vi "Stop.vi"(8 "error in":errorcluster, 11 "WaveformTask in":refnum<class "WaveformTask.lvclass">) -> (0 "error out":errorcluster, 3 "Task out":refnum<class "WaveformTask.lvclass">)   [LabVIEW 2015, in "WaveformTask.lvclass"]
uses:
  WaveformTask.lvclass
  WaveformTask.lvclass/WaveformTask.ctl
  <vilib>/NI/cRIO Wfm/ErrorSelector.ctl
  <vilib>/Utility/error.llb/Error Cluster From Error Code.vi
  <vilib>/rvi/errors/niLvFpgaAdjustHostInterfaceError.vi
  <vilib>/rvi/interface/nirviMethod/nirviMethod.xnode
  DataFIFOs.ctl
  <vilib>/NI/cRIO Wfm/cRIO Wfm.lvlib
  <vilib>/FPGAPlugInAG/Dynamic/niLvFpga_ReadFifo_Dynamic.vi
  <vilib>/rvi/errors/niLvFpgaMergeErrorWithErrorCode.vi
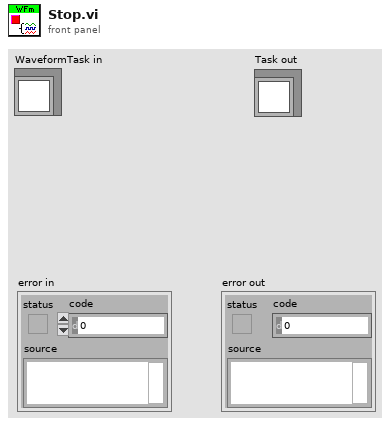
[diagram p1: front panel]
types:
  T1 = typedef "WaveformTask.lvclass/DataFIFOs.ctl" = refnum<k20>
  T2 = typedef "cRIO Wfm.lvlib/ErrorSelector.ctl" = enum16{"Read Timeout", "Module Underflow", "DMA Overflow", "Chan Count", "Run Timeout", "Start Timeout", "Stop Timeout"}
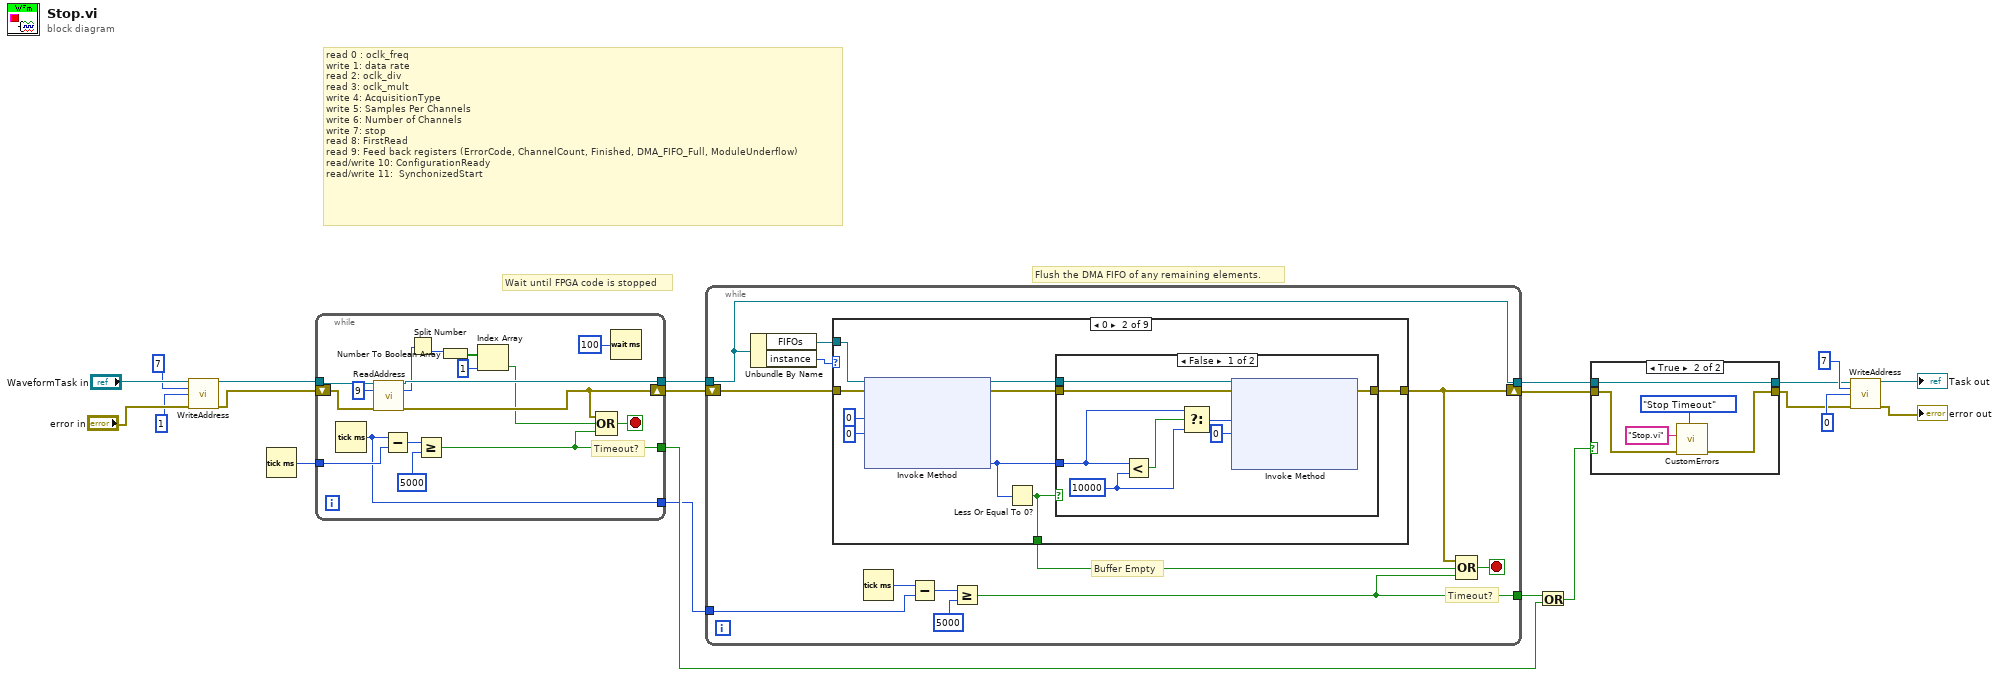
[diagram p0: block diagram]
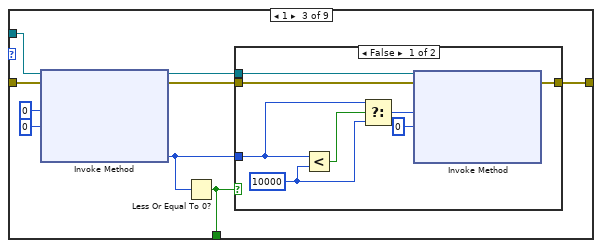
[diagram p4: hidden frame]
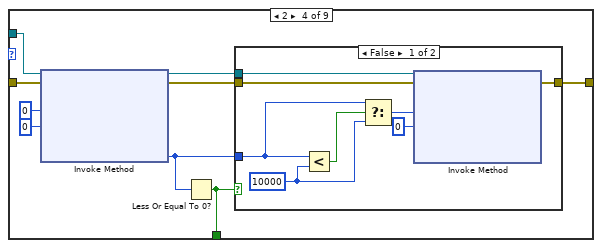
[diagram p6: hidden frame]
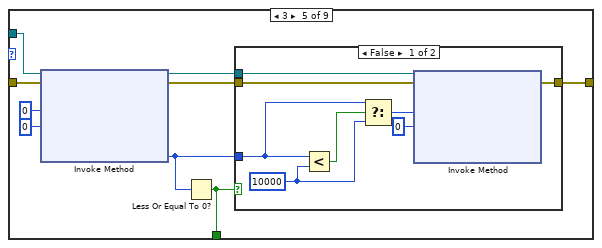
[diagram p8: hidden frame]
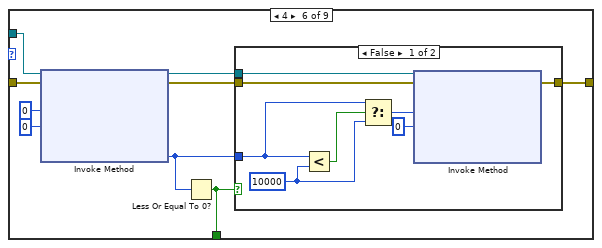
[diagram p10: hidden frame]
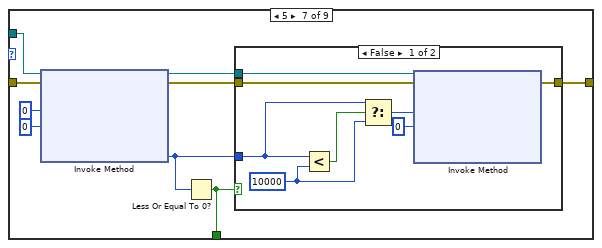
[diagram p12: hidden frame]
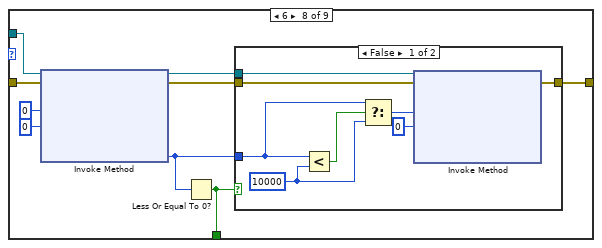
[diagram p14: hidden frame]
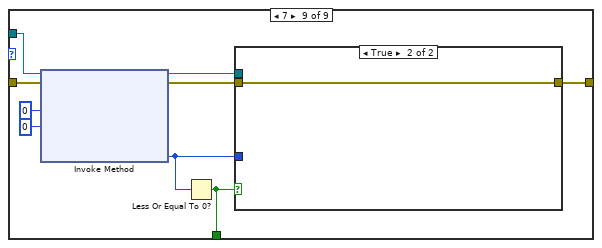
[diagram p16: hidden frame]
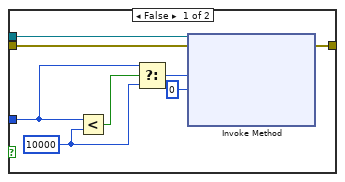
[diagram p17: hidden frame]
diagram:
  # "read 0 : oclk_freq\nwrite 1: data rate\nread 2: oclk_div\nread 3: oclk_mult\nwrite 4: AcquisitionType\nwrite 5: Samples Per Channels\nwrite 6: Number of Channels\nwrite 7: stop\nread 8: FirstRead\nread 9: Feed back registers (ErrorCode, ChannelCount, Finished, DMA_FIFO_Full, ModuleUnderflow)\nread/write 10: ConfigurationReady\nread/write 11:  SynchonizedStart"
  # "Wait until FPGA code is stopped"
  # "Flush the DMA FIFO of any remaining elements."
  n1 = call "WriteAddress.vi"("Task in"="WaveformTask in", "address"=u64 7, "data"=u64 1, "error in (no error)"="error in") -> ("Task out"=w7:refnum<class "WaveformTask.lvclass">, "error out"=w8:errorcluster)  [unwired: 10 in]
  n2 = Tick Count (ms)() -> (millisecond timer value=w17:u32)
  n3 = while {
    tunnel: w7 -> [w31]
    tunnel: [w29] -> w21
    tunnel: w17 -> [w37]
    tunnel: [w33] -> w15
    tunnel: [w32] -> w13
    shift-right: [w27] -> w20
    shift-left: w8 -> [w30]
    stop <- w34 stop-if-true
    # "Timeout?"
    n4 = Tick Count (ms)() -> (millisecond timer value=w32:u32)
    n5 = call "ReadAddress.vi"("Task in"=w31, "address"=u64 9, "error in (no error)"=w30) -> ("Task out"=w29:refnum<class "WaveformTask.lvclass">, "data"=w26:u64, "error out"=w27:errorcluster)  [unwired: 10 in]
    n6 = Subtract(x=w32, y=w37) -> (x-y=w36:u32)
    n7 = Split Number(x=w26) -> (lo(x)=w25:u32)  [unwired: 1 out]
    n8 = Greater Or Equal?(x=w36, y=u32 5000) -> (x >= y?=w33:bool)
    n9 = Number To Boolean Array(number=w25) -> (Boolean array=w24:bool[])
    n10 = Index Array(array=w24, index=1) -> (element=w22:bool)
    n11 = Compound Arithmetic op=OR(w27, w22, w33) -> (w34:bool)
    n12 = Wait (ms)(milliseconds to wait=u32 100) -> ()  [unwired: 1 out]
  }
  n13 = while {
    tunnel: [w39] -> w19
    tunnel: w21 -> [w39]
    tunnel: w13 -> [w44]
    tunnel: [w43] -> w16
    shift-right: [w42] -> w18
    shift-left: w20 -> [w50]
    stop <- w49 stop-if-true
    # "Timeout?"
    # "Buffer Empty"
    n14 = Unbundle By Name(w39) -> ("FIFOs"=w40:T1, "instance"=w41:u8)
    n15 = case shown="0" w41 {
      tunnel: w50 -> [w51 w56 w74 w92 w110 w128 w146 w164 w182]
      tunnel: [_ w54 w72 w90 w108 w126 w144 w162 w180] -> w48
      tunnel: [w51 w53 w71 w89 w107 w125 w143 w161 w179] -> w42
      tunnel: w40 -> [_ w52 w70 w88 w106 w124 w142 w160 w178]
      frame Default {
        # "#TODO error"
      }
      frame 0 {
        n16 = xnode "Invoke Method"("FPGA VI Reference In"=w52, "error in"=w56, "Number of Elements"=u32 0, "Timeout (ms)"=0) -> ("FPGA VI Reference Out"=w60:T1, "error out"=w59:errorcluster, "Elements Remaining"=w55:u32)  [unwired: 1 out]
        n17 = Less Or Equal To 0?(x=w55) -> (x <= 0?=w54:bool)
        n18 = case shown="False" w54 {
          tunnel: w60 -> [w68 _]
          tunnel: w59 -> [w67 w69]
          tunnel: [w65 w69] -> w53
          tunnel: w55 -> [w61 _]
          frame False {
            w63 = u32 10000
            n19 = Less?(x=w61, y=w63) -> (x < y?=w64:bool)
            n20 = Select(t=w61, s=w64, f=w63) -> (s? t:f=w62:u32)
            n21 = xnode "Invoke Method"("FPGA VI Reference In"=w68, "error in"=w67, "Number of Elements"=w62, "Timeout (ms)"=0) -> ("error out"=w65:errorcluster)  [unwired: 3 out]
          }
          frame True {
          }
        }
      }
      frame 1 {
        n22 = xnode "Invoke Method"("FPGA VI Reference In"=w70, "error in"=w74, "Number of Elements"=u32 0, "Timeout (ms)"=0) -> ("FPGA VI Reference Out"=w78:T1, "error out"=w77:errorcluster, "Elements Remaining"=w73:u32)  [unwired: 1 out]
        n23 = Less Or Equal To 0?(x=w73) -> (x <= 0?=w72:bool)
        n24 = case shown="False" w72 {
          tunnel: w78 -> [w86 _]
          tunnel: w77 -> [w85 w87]
          tunnel: [w83 w87] -> w71
          tunnel: w73 -> [w79 _]
          frame False {
            w81 = u32 10000
            n25 = Less?(x=w79, y=w81) -> (x < y?=w82:bool)
            n26 = Select(t=w79, s=w82, f=w81) -> (s? t:f=w80:u32)
            n27 = xnode "Invoke Method"("FPGA VI Reference In"=w86, "error in"=w85, "Number of Elements"=w80, "Timeout (ms)"=0) -> ("error out"=w83:errorcluster)  [unwired: 3 out]
          }
          frame True {
          }
        }
      }
      frame 2 {
        n28 = xnode "Invoke Method"("FPGA VI Reference In"=w88, "error in"=w92, "Number of Elements"=u32 0, "Timeout (ms)"=0) -> ("FPGA VI Reference Out"=w96:T1, "error out"=w95:errorcluster, "Elements Remaining"=w91:u32)  [unwired: 1 out]
        n29 = Less Or Equal To 0?(x=w91) -> (x <= 0?=w90:bool)
        n30 = case shown="False" w90 {
          tunnel: w96 -> [w104 _]
          tunnel: w95 -> [w103 w105]
          tunnel: [w101 w105] -> w89
          tunnel: w91 -> [w97 _]
          frame False {
            w99 = u32 10000
            n31 = Less?(x=w97, y=w99) -> (x < y?=w100:bool)
            n32 = Select(t=w97, s=w100, f=w99) -> (s? t:f=w98:u32)
            n33 = xnode "Invoke Method"("FPGA VI Reference In"=w104, "error in"=w103, "Number of Elements"=w98, "Timeout (ms)"=0) -> ("error out"=w101:errorcluster)  [unwired: 3 out]
          }
          frame True {
          }
        }
      }
      frame 3 {
        n34 = xnode "Invoke Method"("FPGA VI Reference In"=w106, "error in"=w110, "Number of Elements"=u32 0, "Timeout (ms)"=0) -> ("FPGA VI Reference Out"=w114:T1, "error out"=w113:errorcluster, "Elements Remaining"=w109:u32)  [unwired: 1 out]
        n35 = Less Or Equal To 0?(x=w109) -> (x <= 0?=w108:bool)
        n36 = case shown="False" w108 {
          tunnel: w114 -> [w122 _]
          tunnel: w113 -> [w121 w123]
          tunnel: [w119 w123] -> w107
          tunnel: w109 -> [w115 _]
          frame False {
            w117 = u32 10000
            n37 = Less?(x=w115, y=w117) -> (x < y?=w118:bool)
            n38 = Select(t=w115, s=w118, f=w117) -> (s? t:f=w116:u32)
            n39 = xnode "Invoke Method"("FPGA VI Reference In"=w122, "error in"=w121, "Number of Elements"=w116, "Timeout (ms)"=0) -> ("error out"=w119:errorcluster)  [unwired: 3 out]
          }
          frame True {
          }
        }
      }
      frame 4 {
        n40 = xnode "Invoke Method"("FPGA VI Reference In"=w124, "error in"=w128, "Number of Elements"=u32 0, "Timeout (ms)"=0) -> ("FPGA VI Reference Out"=w132:T1, "error out"=w131:errorcluster, "Elements Remaining"=w127:u32)  [unwired: 1 out]
        n41 = Less Or Equal To 0?(x=w127) -> (x <= 0?=w126:bool)
        n42 = case shown="False" w126 {
          tunnel: w132 -> [w140 _]
          tunnel: w131 -> [w139 w141]
          tunnel: [w137 w141] -> w125
          tunnel: w127 -> [w133 _]
          frame False {
            w135 = u32 10000
            n43 = Less?(x=w133, y=w135) -> (x < y?=w136:bool)
            n44 = Select(t=w133, s=w136, f=w135) -> (s? t:f=w134:u32)
            n45 = xnode "Invoke Method"("FPGA VI Reference In"=w140, "error in"=w139, "Number of Elements"=w134, "Timeout (ms)"=0) -> ("error out"=w137:errorcluster)  [unwired: 3 out]
          }
          frame True {
          }
        }
      }
      frame 5 {
        n46 = xnode "Invoke Method"("FPGA VI Reference In"=w142, "error in"=w146, "Number of Elements"=u32 0, "Timeout (ms)"=0) -> ("FPGA VI Reference Out"=w150:T1, "error out"=w149:errorcluster, "Elements Remaining"=w145:u32)  [unwired: 1 out]
        n47 = Less Or Equal To 0?(x=w145) -> (x <= 0?=w144:bool)
        n48 = case shown="False" w144 {
          tunnel: w150 -> [w158 _]
          tunnel: w149 -> [w157 w159]
          tunnel: [w155 w159] -> w143
          tunnel: w145 -> [w151 _]
          frame False {
            w153 = u32 10000
            n49 = Less?(x=w151, y=w153) -> (x < y?=w154:bool)
            n50 = Select(t=w151, s=w154, f=w153) -> (s? t:f=w152:u32)
            n51 = xnode "Invoke Method"("FPGA VI Reference In"=w158, "error in"=w157, "Number of Elements"=w152, "Timeout (ms)"=0) -> ("error out"=w155:errorcluster)  [unwired: 3 out]
          }
          frame True {
          }
        }
      }
      frame 6 {
        n52 = xnode "Invoke Method"("FPGA VI Reference In"=w160, "error in"=w164, "Number of Elements"=u32 0, "Timeout (ms)"=0) -> ("FPGA VI Reference Out"=w168:T1, "error out"=w167:errorcluster, "Elements Remaining"=w163:u32)  [unwired: 1 out]
        n53 = Less Or Equal To 0?(x=w163) -> (x <= 0?=w162:bool)
        n54 = case shown="False" w162 {
          tunnel: w168 -> [w176 _]
          tunnel: w167 -> [w175 w177]
          tunnel: [w173 w177] -> w161
          tunnel: w163 -> [w169 _]
          frame False {
            w171 = u32 10000
            n55 = Less?(x=w169, y=w171) -> (x < y?=w172:bool)
            n56 = Select(t=w169, s=w172, f=w171) -> (s? t:f=w170:u32)
            n57 = xnode "Invoke Method"("FPGA VI Reference In"=w176, "error in"=w175, "Number of Elements"=w170, "Timeout (ms)"=0) -> ("error out"=w173:errorcluster)  [unwired: 3 out]
          }
          frame True {
          }
        }
      }
      frame 7 {
        n58 = xnode "Invoke Method"("FPGA VI Reference In"=w178, "error in"=w182, "Number of Elements"=u32 0, "Timeout (ms)"=0) -> ("FPGA VI Reference Out"=w186:T1, "error out"=w185:errorcluster, "Elements Remaining"=w181:u32)  [unwired: 1 out]
        n59 = Less Or Equal To 0?(x=w181) -> (x <= 0?=w180:bool)
        n60 = case shown="True" w180 {
          tunnel: w186 -> [w194 _]
          tunnel: w185 -> [w193 w195]
          tunnel: [w191 w195] -> w179
          tunnel: w181 -> [w187 _]
          frame False {
            w189 = u32 10000
            n61 = Less?(x=w187, y=w189) -> (x < y?=w190:bool)
            n62 = Select(t=w187, s=w190, f=w189) -> (s? t:f=w188:u32)
            n63 = xnode "Invoke Method"("FPGA VI Reference In"=w194, "error in"=w193, "Number of Elements"=w188, "Timeout (ms)"=0) -> ("error out"=w191:errorcluster)  [unwired: 3 out]
          }
          frame True {
          }
        }
      }
    }
    n64 = Tick Count (ms)() -> (millisecond timer value=w45:u32)
    n65 = Subtract(x=w45, y=w44) -> (x-y=w46:u32)
    n66 = Greater Or Equal?(x=w46, y=u32 5000) -> (x >= y?=w43:bool)
    n67 = Compound Arithmetic op=OR(w42, w48, w43) -> (w49:bool)
  }
  n68 = Or(x=w16, y=w15) -> (x .or. y?=w14:bool)
  n69 = case shown="True" w14 {
    tunnel: [w197 w202] -> w4
    tunnel: w19 -> [w197 w202]
    tunnel: w18 -> [w196 w201]
    tunnel: [w196 w200] -> w2
    frame False {
    }
    frame True {
      n70 = call <vilib>:"CustomErrors.vi"("Error Selector"=ErrorSelector."Stop Timeout", "error in"=w201, "Calling VI"="Stop.vi") -> ("error out"=w200:errorcluster)  [unwired: 8 in]
    }
  }
  n71 = call "WriteAddress.vi"("Task in"=w4, "address"=u64 7, "data"=u64 0, "error in (no error)"=w2) -> ("Task out"=→"Task out":refnum<class "WaveformTask.lvclass">, "error out"=→"error out":errorcluster)  [unwired: 10 in]
